vi "Configure Output Range Core.vi"(6 "range (0.0)":dbl format="%^.2e", 8 "error in (no error)":errorcluster, 9 "range type (Voltage)":i32(ring)=1 items=["Voltage"=1, "Current"=0], 10 "channel name (\"CHANNEL1\")":string="CHANNEL1", 11 "IVI_DCPwr in":refnum<class "IVI_DCPwr.lvclass">) -> (0 "error out":errorcluster, 3 "IVI_DCPwr out":refnum<class "IVI_DCPwr.lvclass">)   [LabVIEW 2015, in "IVI_DCPwr.lvlib" / "IVI_DCPwr.lvclass"]
doc: "Configures the power supply's output range on a channel. You specify whether you want to configure the voltage or current range, and the value to which to set the range.\n\nNotes:\n\n1) Setting a voltage range can invalidate a previously configured current range.\n\n2) Setting a current range can invalidate a previously configured voltage range."
uses:
  IVI_DCPwr.lvclass
  IVI_DCPwr.lvclass/IVI_DCPwr.ctl
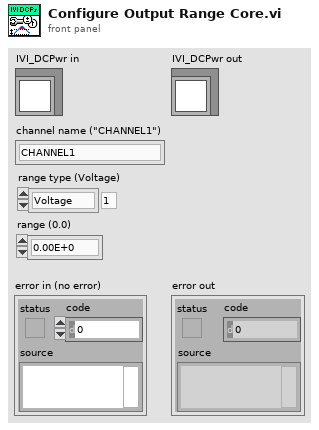
[diagram p1: front panel]
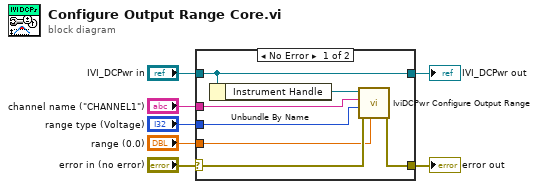
[diagram p0: block diagram]
diagram:
  n1 = case shown="No Error" "error in (no error)" {
    selector: "error in (no error)" -> [w12 w16]
    tunnel: [w11 w16] -> w6
    tunnel: [w14 w15] -> w4
    tunnel: "IVI_DCPwr in" -> [w14 w15]
    tunnel: "channel name (\"CHANNEL1\")" -> [w10 _]
    tunnel: "range type (Voltage)" -> [w9 _]
    tunnel: "range (0.0)" -> [w8 _]
    frame No Error {
      n2 = Unbundle By Name(w14) -> ("Instrument Handle"=w13:refnum<k15>)
      n3 = call <vilib>:"IviDCPwr Configure Output Range.vi"("range (0.0)"=w8, "error in (no error)"=w12, "range type (Voltage)"=w9, "channel name (\"CHANNEL1\")"=w10, "instrument handle"=w13) -> ("error out"=w11:errorcluster)  [unwired: 5 in, 1 out]
    }
    frame Error {
    }
  }
  "error out" <- w6
  "IVI_DCPwr out" <- w4
